vi "GE 5565PIORC.Registers.PCI Command.Interrupt Disable.Get.vi"(8 "error in (no error)":errorcluster, 11 "GE 5565PIORC in":refnum<class "GE 5565PIORC.lvclass">) -> (0 "error out":errorcluster, 2 "Interrupt Disable":bool, 3 "GE 5565PIORC out":refnum<class "GE 5565PIORC.lvclass">)   [LabVIEW 2024, in "GE 5565PIORC.lvclass"]
doc: "When set (1), this bit disables the Reflective Memory from asserting its interrupt pin. When not set (0), interrupts are generated normally."
uses:
  GE 5565PIORC.lvclass
  GE 5565PIORC.Registers.PCI Configuration.ctl
  GE 5565PIORC.lvclass/GE 5565PIORC.ctl
  Methods/GE 5565PIORC.Bit Manipulation.Get Bit (U16).vi
  GE 5565PIORC.Registers.PCI Configuration.Read (U16).vi
  Methods/GE 5565PIORC.Registers.Read.vi
  Methods/GE 5565PIORC.Registers.Read (U16).vi
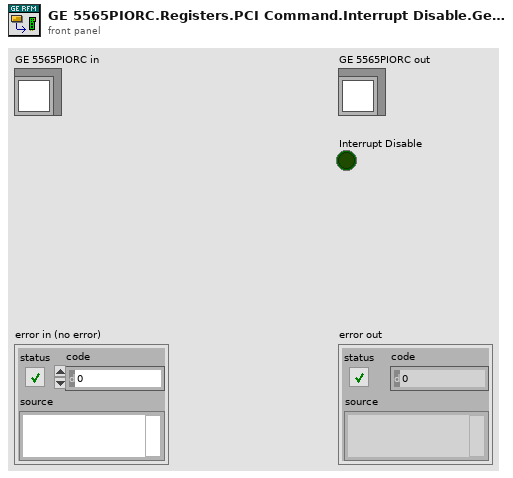
[diagram p1: front panel]
types:
  T1 = typedef "GE 5565PIORC.lvclass/GE 5565PIORC.Registers.PCI Configuration.ctl" = u32
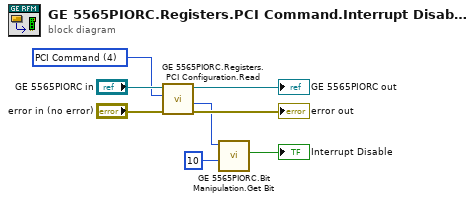
[diagram p0: block diagram]
diagram:
  w1 = T1 4 items=["PCI Configuration ID"=0, "PCI Command"=4, "PCI Status"=6, "PCI Revision ID"=8, "PCI Class Code"=9, "PCI Cache Line Size"=12, "PCI Latency Timer"=13, "PCI Header Type"=14, "PCI Built-in Self Test"=15, "PCIBAR0"=16, "PCIBAR1"=20, "PCIBAR2"=24, "PCIBAR3"=28, "PCIBAR4"=32, "PCIBAR5"=36, "PCI Cardbus CIS Pointer"=40, "PCI Subsystem Vendor ID"=44, "PCI Subsystem ID"=46, "PCI Expansion ROM Base"=48, "Capability Pointer"=52, "PCI Interrupt Line"=60, "PCI Interrupt Pin"=61, "PCI Min_Gnt"=62, "PCI Max_Lat"=63] ("Register")
  n1 = call-poly "GE 5565PIORC.Registers.PCI Configuration.Read.vi"("error in (no error)"="error in (no error)", "Register"=w1, "GE 5565PIORC in"="GE 5565PIORC in") -> ("error out"=→"error out":errorcluster, "Value"=w4:u16, "GE 5565PIORC out"=→"GE 5565PIORC out":refnum<class "GE 5565PIORC.lvclass">)  [unwired: 6 in]
  n2 = call-poly "GE 5565PIORC.Bit Manipulation.Get Bit.vi"("bit index"=10, "packed value in"=w4) -> ("bit"=→"Interrupt Disable":bool)  [unwired: 8 in, 1 out]
